vi "assert_console_close.vi"(8 "error in (no error)":errorcluster, 11 "console.provider in":refnum<class "console.provider.lvclass">) -> (0 "error out":errorcluster)   [LabVIEW 2021, in "console.provider.lvclass"]
uses:
  console.provider.lvclass
  console.provider.lvclass/console.provider.ctl
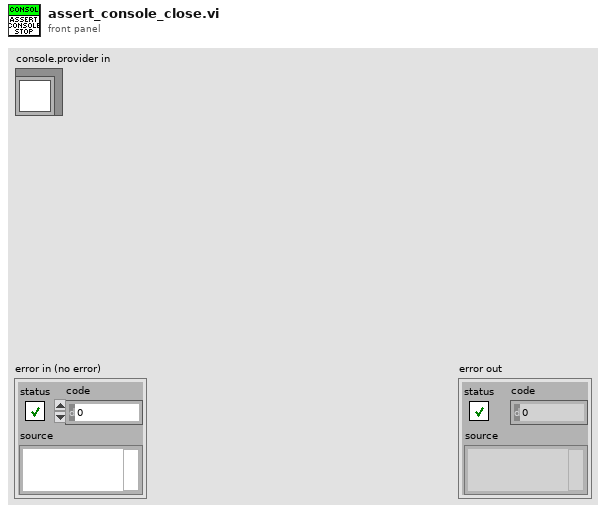
[diagram p1: front panel]
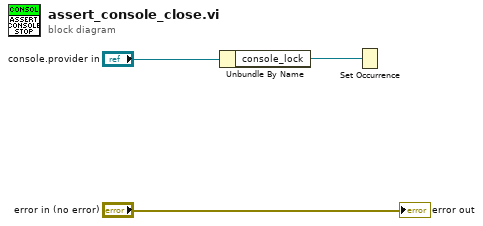
[diagram p0: block diagram]
diagram:
  n1 = Unbundle By Name("console.provider in") -> ("console_lock"=w1:refnum<k4>)
  n2 = Set Occurrence(w1) -> ()
  "error out" <- "error in (no error)"
